vi "Thorlabs_TDC001.ProcCases.vi"(0 "i ref in":refnum<vi>, 1 "selector":string, 2 "Data":T1, 3 "call cluster":T2={"Object"="", "Selector"="", "CallType"=enum."synchronous", "Async Object"="", "Async Selector"="", "Data Descriptor"="", "Data"=[], "Error #"=0, "Expire"=0}, 5 "error in (no error)":errorcluster) -> (14 "i ref out":refnum<vi>, 17 "answer cluster":T2={"Object"="", "Selector"="", "CallType"=enum."synchronous", "Async Object"="", "Async Selector"="", "Data Descriptor"="", "Data"=[], "Error #"=0, "Expire"=0}, 19 "error out":errorcluster)   [LabVIEW 2014, in "Thorlabs_TDC001.lvlib"]
doc: "This method is called by a process from within the default case in the event loop. The methods of a class that are linked to events will be called from THIS method. Add your code here."
uses:
  Thorlabs_TDC001.lvlib
  CS_Core/CSSystem/CoreDefs/CoreDefs.call_type.ctl
  CS_Core/BaseProcess/BaseProcess.descriptor string definition.ctl
  CS_Core/CSSystem/CoreDefs/CoreDefs.rawDataType.ctl
  CS_Core/CSSystem/CoreLib/CoreLib.string 2 byte array.vi
  CS_Core/CSSystem/CoreLib/CoreLib.double 2 byte array.vi
  CS_Core/CSSystem/CoreLib/CoreLib.byte array 2 double.vi
  CS_Core/CSSystem/CoreLib/CoreLib.lvlib
  CS_Core/BaseProcess/BaseProcess.lvlib
  CS_Core/CSApplicationBaseClasses/DeviceBase/DeviceBase.lvlib
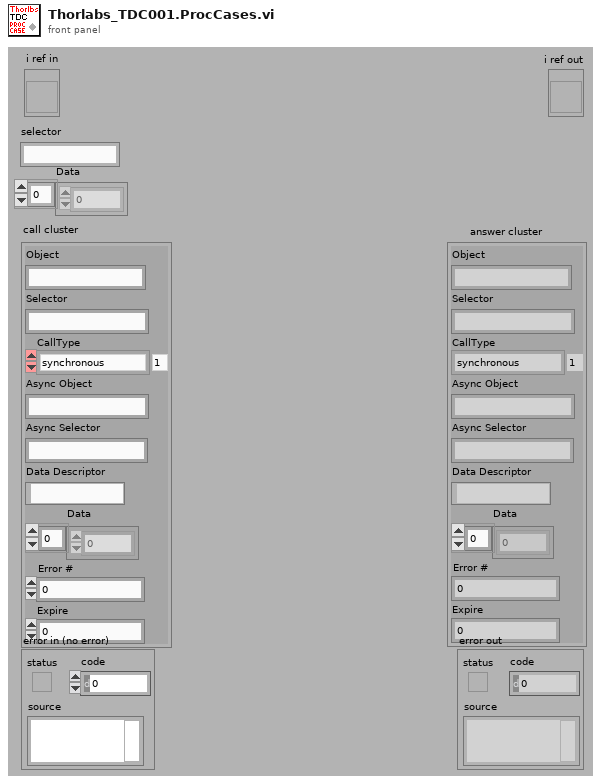
[diagram p1: front panel]
types:
  T1 = typedef "CoreDefs.rawDataType.ctl" = i8[]
  T2 = typedef "CoreDefs.call_type.ctl" = cluster{"Object":string, "Selector":string, "CallType":enum16{"simple", "synchronous", "asynchronous"}, "Async Object":string, "Async Selector":string, "Data Descriptor":T3, "Data":T1, "Error #":i32, "Expire":u32}
  T3 = typedef "BaseProcess.lvlib/BaseProcess.descriptor string definition.ctl" = string
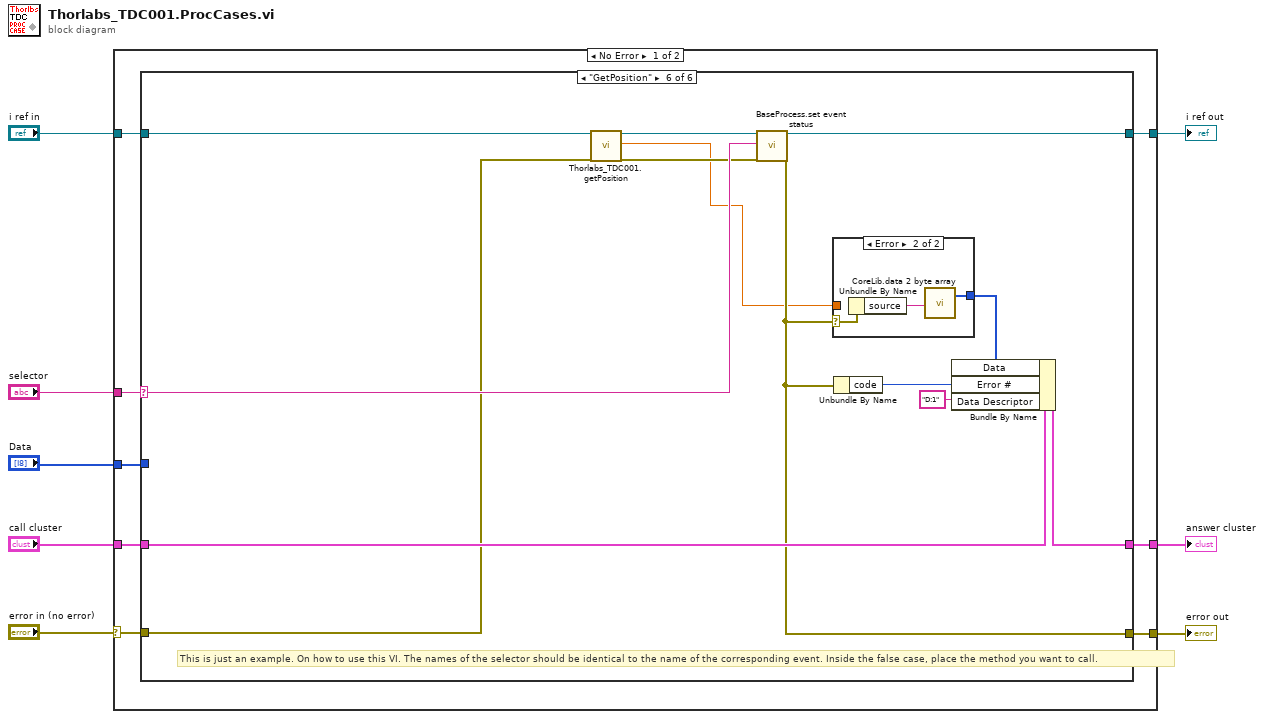
[diagram p0: block diagram]
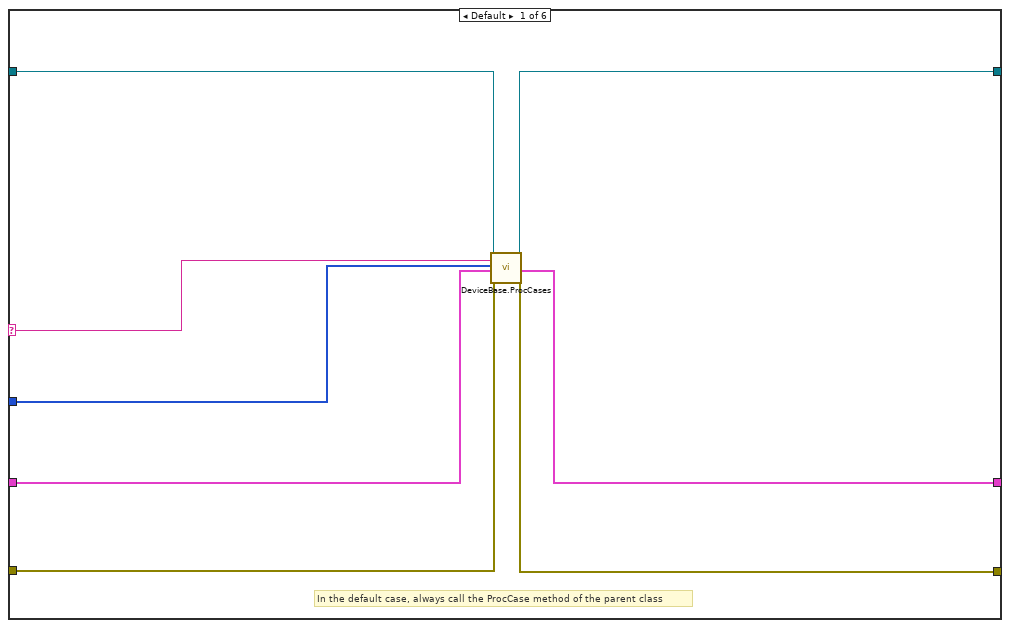
[diagram p2: hidden frame]
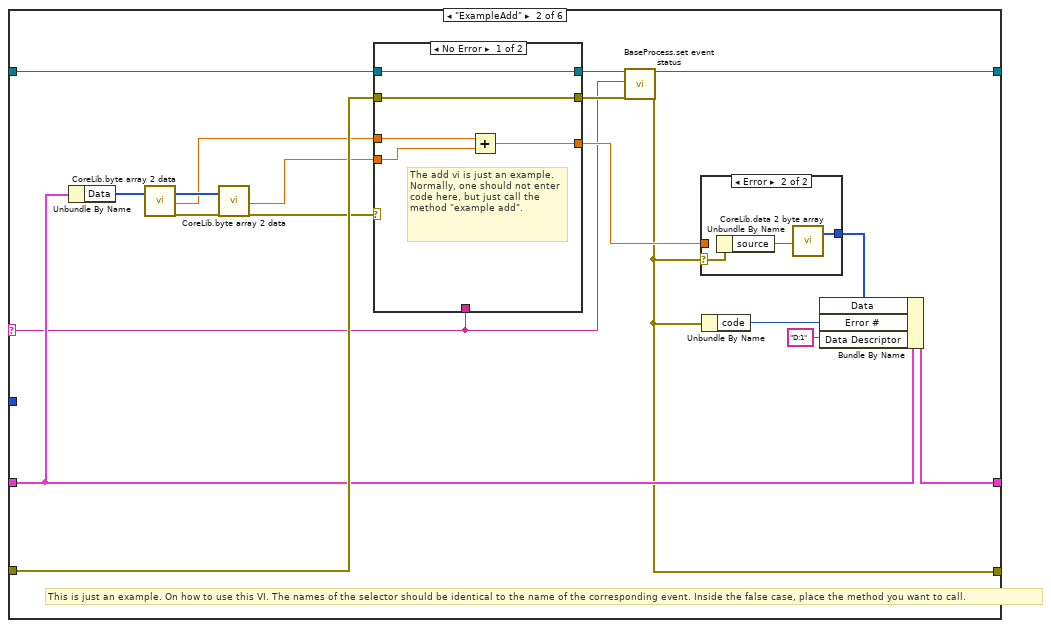
[diagram p3: hidden frame]
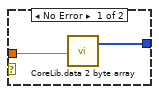
[diagram p4: hidden frame]
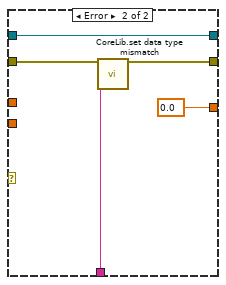
[diagram p5: hidden frame]
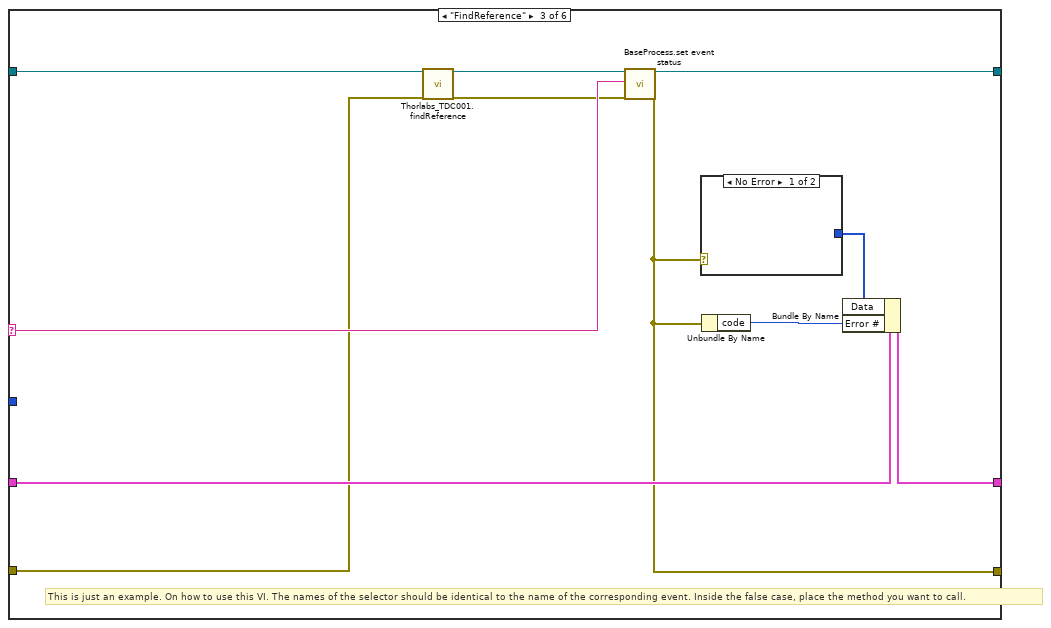
[diagram p6: hidden frame]
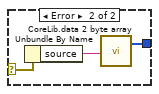
[diagram p7: hidden frame]
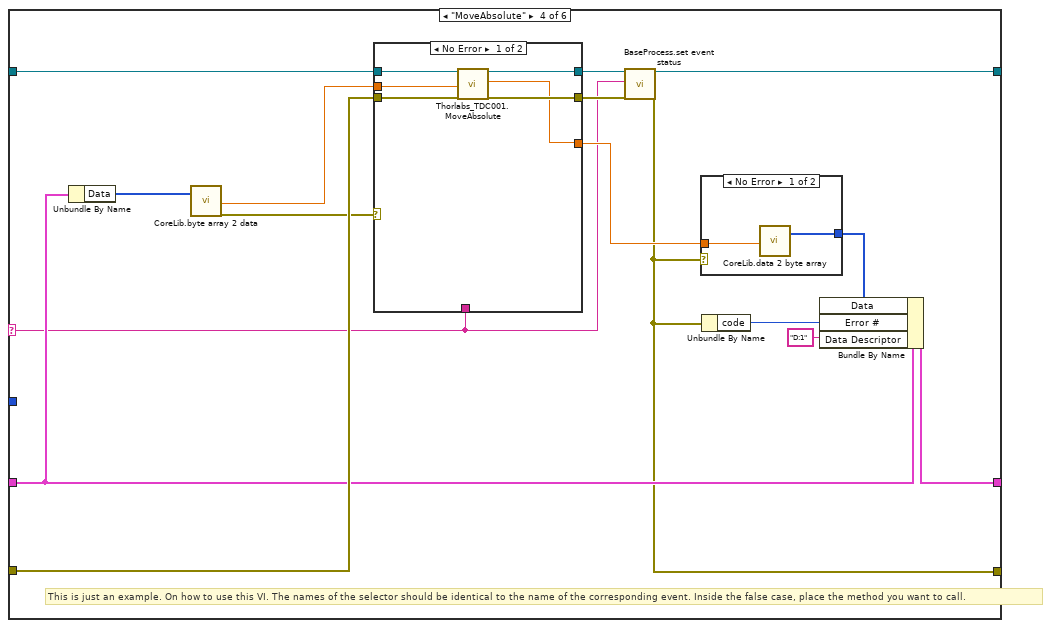
[diagram p8: hidden frame]
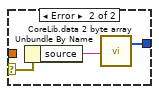
[diagram p9: hidden frame]
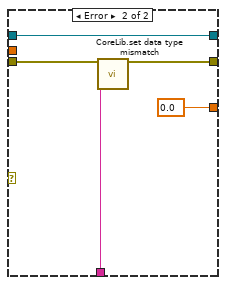
[diagram p10: hidden frame]
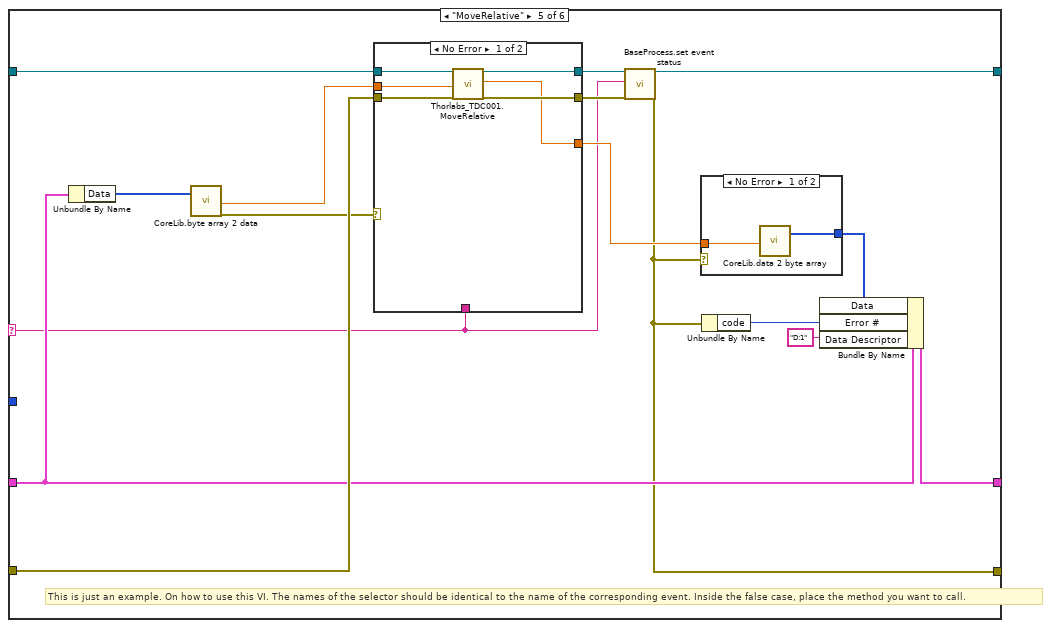
[diagram p11: hidden frame]
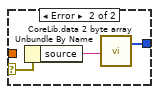
[diagram p12: hidden frame]
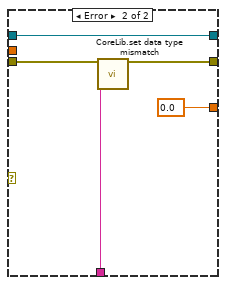
[diagram p13: hidden frame]
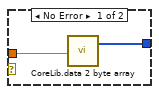
[diagram p14: hidden frame]
diagram:
  n1 = case shown="No Error" "error in (no error)" {
    selector: "error in (no error)" -> [w9 w155]
    tunnel: "selector" -> [w16 _]
    tunnel: [w15 w156] -> w7
    tunnel: "Data" -> [w14 _]
    tunnel: "call cluster" -> [w13 w156]
    tunnel: "i ref in" -> [w12 w157]
    tunnel: [w11 w157] -> w3
    tunnel: [w10 w155] -> w2
    frame No Error {
      n2 = case shown="\"GetPosition\"" w16 {
        selector: w16 -> [w19 w33 w64 w78 w110 w144]
        tunnel: w14 -> [w17 _ _ _ _ _]
        tunnel: w12 -> [w18 w43 w62 w88 w120 w141]
        tunnel: [w24 w32 w63 w77 w109 w143] -> w11
        tunnel: w13 -> [w20 w39 w68 w84 w116 w148]
        tunnel: [w21 w38 w67 w83 w115 w147] -> w15
        tunnel: w9 -> [w23 w42 w60 w87 w119 w140]
        tunnel: [w22 w34 w65 w79 w111 w145] -> w10
        frame Default {
          # "In the default case, always call the ProcCase method of the parent class"
          n3 = call "DeviceBase.ProcCases.vi"("i ref in"=w18, "selector"=w19, "Data"=w17, "call cluster"=w20, "error in (no error)"=w23) -> ("i ref out"=w24:refnum<vi>, "answer cluster"=w21:T2, "error out"=w22:errorcluster)  [unwired: 12 in]
        }
        frame "ExampleAdd" {
          # "This is just an example. On how to use this VI. The names of the selector should be identical to the name of the corresponding event. Inside the false case, place the method you want to call."
          n4 = Unbundle By Name(w39) -> ("Data"=w30:T1)
          n5 = call-poly "CoreLib.byte array 2 data.vi"("byteArray"=w30) -> ("byteArray out"=w28:T1, "d64"=w26:dbl, "error out"=w29:errorcluster)  [unwired: 16 in]
          n6 = call-poly "CoreLib.byte array 2 data.vi"("byteArray"=w28, "error in (no error)"=w29) -> ("d64"=w25:dbl, "error out"=w27:errorcluster)  [unwired: 15 in, 1 out]
          n7 = case shown="No Error" w27 {
            tunnel: [w50 w58] -> w36
            tunnel: w43 -> [w50 w58]
            tunnel: w42 -> [w51 w57]
            tunnel: [w51 w56] -> w35
            tunnel: w25 -> [w53 _]
            tunnel: [w52 0.0] -> w41
            tunnel: w33 -> [_ w54]
            tunnel: w26 -> [w49 _]
            frame No Error {
              # "The add vi is just an example. Normally, one should not enter code here, but just call the method \"example add\"."
              n8 = Add(x=w49, y=w53) -> (x+y=w52:dbl)
            }
            frame Error {
              n9 = call "CoreLib.set data type mismatch.vi"("error in (no error)"=w57, "error source"=w54) -> ("error out"=w56:errorcluster)  [unwired: 17 in]
            }
          }
          n10 = call "BaseProcess.set event status.vi"("i ref in"=w36, "EventStatus"=w33, "error in (no error)"=w35) -> ("i ref out"=w32:refnum<vi>, "error out"=w34:errorcluster)  [unwired: 14 in, 1 out]
          n11 = case shown="Error" w34 {
            selector: w34 -> [_ w48]
            tunnel: [w44 w47] -> w37
            tunnel: w41 -> [w45 _]
            frame No Error {
              n12 = call-poly "CoreLib.data 2 byte array.vi"("f64"=w45) -> ("byteArray out"=w44:T1)  [unwired: 18 in]
            }
            frame Error {
              n13 = Unbundle By Name(w48) -> ("source"=w46:string)
              n14 = call-poly "CoreLib.data 2 byte array.vi"("string"=w46) -> ("byteArray out"=w47:T1)  [unwired: 18 in]
            }
          }
          n15 = Unbundle By Name(w34) -> ("code"=w40:i32)
          n16 = Bundle By Name(cluster=w39, "Data"=w37, "Error #"=w40, "Data Descriptor"="D:1") -> (w38:T2)
        }
        frame "FindReference" {
          # "This is just an example. On how to use this VI. The names of the selector should be identical to the name of the corresponding event. Inside the false case, place the method you want to call."
          n17 = call "Thorlabs_TDC001.findReference.vi"("i ref in"=w62, "error in (no error)"=w60) -> ("i ref out"=w61:refnum<vi>, "error out"=w59:errorcluster)  [unwired: 16 in]
          n18 = call "BaseProcess.set event status.vi"("i ref in"=w61, "EventStatus"=w64, "error in (no error)"=w59) -> ("i ref out"=w63:refnum<vi>, "error out"=w65:errorcluster)  [unwired: 14 in, 1 out]
          n19 = case shown="No Error" w65 {
            selector: w65 -> [_ w72]
            tunnel: [_ w71] -> w66
            frame No Error {
            }
            frame Error {
              n20 = Unbundle By Name(w72) -> ("source"=w70:string)
              n21 = call-poly "CoreLib.data 2 byte array.vi"("string"=w70) -> ("byteArray out"=w71:T1)  [unwired: 18 in]
            }
          }
          n22 = Unbundle By Name(w65) -> ("code"=w69:i32)
          n23 = Bundle By Name(cluster=w68, "Data"=w66, "Error #"=w69) -> (w67:T2)
        }
        frame "MoveAbsolute" {
          # "This is just an example. On how to use this VI. The names of the selector should be identical to the name of the corresponding event. Inside the false case, place the method you want to call."
          n24 = Unbundle By Name(w84) -> ("Data"=w75:T1)
          n25 = call-poly "CoreLib.byte array 2 data.vi"("byteArray"=w75) -> ("d64"=w73:dbl, "error out"=w74:errorcluster)  [unwired: 16 in, 1 out]
          n26 = case shown="No Error" w74 {
            tunnel: [w98 w104] -> w81
            tunnel: w88 -> [w99 w104]
            tunnel: w87 -> [w97 w103]
            tunnel: [w96 w102] -> w80
            tunnel: [w94 0.0] -> w86
            tunnel: w78 -> [_ w100]
            tunnel: w73 -> [w95 _]
            frame No Error {
              n27 = call "Thorlabs_TDC001.MoveAbsolute.vi"("i ref in"=w99, "fAbsPos in"=w95, "error in (no error)"=w97) -> ("i ref out"=w98:refnum<vi>, "fAbsPos out"=w94:sgl, "error out"=w96:errorcluster)  [unwired: 14 in]
            }
            frame Error {
              n28 = call "CoreLib.set data type mismatch.vi"("error in (no error)"=w103, "error source"=w100) -> ("error out"=w102:errorcluster)  [unwired: 17 in]
            }
          }
          n29 = call "BaseProcess.set event status.vi"("i ref in"=w81, "EventStatus"=w78, "error in (no error)"=w80) -> ("i ref out"=w77:refnum<vi>, "error out"=w79:errorcluster)  [unwired: 14 in, 1 out]
          n30 = case shown="No Error" w79 {
            selector: w79 -> [_ w93]
            tunnel: [w89 w92] -> w82
            tunnel: w86 -> [w90 _]
            frame No Error {
              n31 = call-poly "CoreLib.data 2 byte array.vi"("f64"=w90) -> ("byteArray out"=w89:T1)  [unwired: 18 in]
            }
            frame Error {
              n32 = Unbundle By Name(w93) -> ("source"=w91:string)
              n33 = call-poly "CoreLib.data 2 byte array.vi"("string"=w91) -> ("byteArray out"=w92:T1)  [unwired: 18 in]
            }
          }
          n34 = Unbundle By Name(w79) -> ("code"=w85:i32)
          n35 = Bundle By Name(cluster=w84, "Data"=w82, "Error #"=w85, "Data Descriptor"="D:1") -> (w83:T2)
        }
        frame "MoveRelative" {
          # "This is just an example. On how to use this VI. The names of the selector should be identical to the name of the corresponding event. Inside the false case, place the method you want to call."
          n36 = Unbundle By Name(w116) -> ("Data"=w107:T1)
          n37 = call-poly "CoreLib.byte array 2 data.vi"("byteArray"=w107) -> ("d64"=w105:dbl, "error out"=w106:errorcluster)  [unwired: 16 in, 1 out]
          n38 = case shown="No Error" w106 {
            tunnel: [w130 w136] -> w113
            tunnel: w120 -> [w131 w136]
            tunnel: w119 -> [w129 w135]
            tunnel: [w128 w134] -> w112
            tunnel: [w126 0.0] -> w118
            tunnel: w110 -> [_ w132]
            tunnel: w105 -> [w127 _]
            frame No Error {
              n39 = call "Thorlabs_TDC001.MoveRelative.vi"("i ref in"=w131, "fRelDist in"=w127, "error in (no error)"=w129) -> ("i ref out"=w130:refnum<vi>, "fRelDist out"=w126:sgl, "error out"=w128:errorcluster)  [unwired: 14 in]
            }
            frame Error {
              n40 = call "CoreLib.set data type mismatch.vi"("error in (no error)"=w135, "error source"=w132) -> ("error out"=w134:errorcluster)  [unwired: 17 in]
            }
          }
          n41 = call "BaseProcess.set event status.vi"("i ref in"=w113, "EventStatus"=w110, "error in (no error)"=w112) -> ("i ref out"=w109:refnum<vi>, "error out"=w111:errorcluster)  [unwired: 14 in, 1 out]
          n42 = case shown="No Error" w111 {
            selector: w111 -> [_ w125]
            tunnel: [w121 w124] -> w114
            tunnel: w118 -> [w122 _]
            frame No Error {
              n43 = call-poly "CoreLib.data 2 byte array.vi"("f64"=w122) -> ("byteArray out"=w121:T1)  [unwired: 18 in]
            }
            frame Error {
              n44 = Unbundle By Name(w125) -> ("source"=w123:string)
              n45 = call-poly "CoreLib.data 2 byte array.vi"("string"=w123) -> ("byteArray out"=w124:T1)  [unwired: 18 in]
            }
          }
          n46 = Unbundle By Name(w111) -> ("code"=w117:i32)
          n47 = Bundle By Name(cluster=w116, "Data"=w114, "Error #"=w117, "Data Descriptor"="D:1") -> (w115:T2)
        }
        frame "GetPosition" {
          # "This is just an example. On how to use this VI. The names of the selector should be identical to the name of the corresponding event. Inside the false case, place the method you want to call."
          n48 = call "Thorlabs_TDC001.getPosition.vi"("i ref in"=w141, "error in (no error)"=w140) -> ("i ref out"=w138:refnum<vi>, "fPos out"=w137:sgl, "error out"=w139:errorcluster)  [unwired: 15 in]
          n49 = call "BaseProcess.set event status.vi"("i ref in"=w138, "EventStatus"=w144, "error in (no error)"=w139) -> ("i ref out"=w143:refnum<vi>, "error out"=w145:errorcluster)  [unwired: 14 in, 1 out]
          n50 = case shown="Error" w145 {
            selector: w145 -> [_ w154]
            tunnel: [w150 w153] -> w146
            tunnel: w137 -> [w151 _]
            frame No Error {
              n51 = call-poly "CoreLib.data 2 byte array.vi"("f64"=w151) -> ("byteArray out"=w150:T1)  [unwired: 18 in]
            }
            frame Error {
              n52 = Unbundle By Name(w154) -> ("source"=w152:string)
              n53 = call-poly "CoreLib.data 2 byte array.vi"("string"=w152) -> ("byteArray out"=w153:T1)  [unwired: 18 in]
            }
          }
          n54 = Unbundle By Name(w145) -> ("code"=w149:i32)
          n55 = Bundle By Name(cluster=w148, "Data"=w146, "Error #"=w149, "Data Descriptor"="D:1") -> (w147:T2)
        }
      }
    }
    frame Error {
    }
  }
  "answer cluster" <- w7
  "i ref out" <- w3
  "error out" <- w2
